vi "SP.vi"   [LabVIEW 2016]
uses:
  <vilib>/ULx/Create Channel.llb/ULx Create Channel (AI-Voltage-Basic).vi
  <vilib>/ULx/Timing.llb/ULx Timing (Sample Clock).vi
  <vilib>/ULx/Read.llb/ULx Read (Analog 1D Wfm NChan NSamp).vi
  <vilib>/Waveform/WDTOps.llb/WDT Index Channel DBL.vi
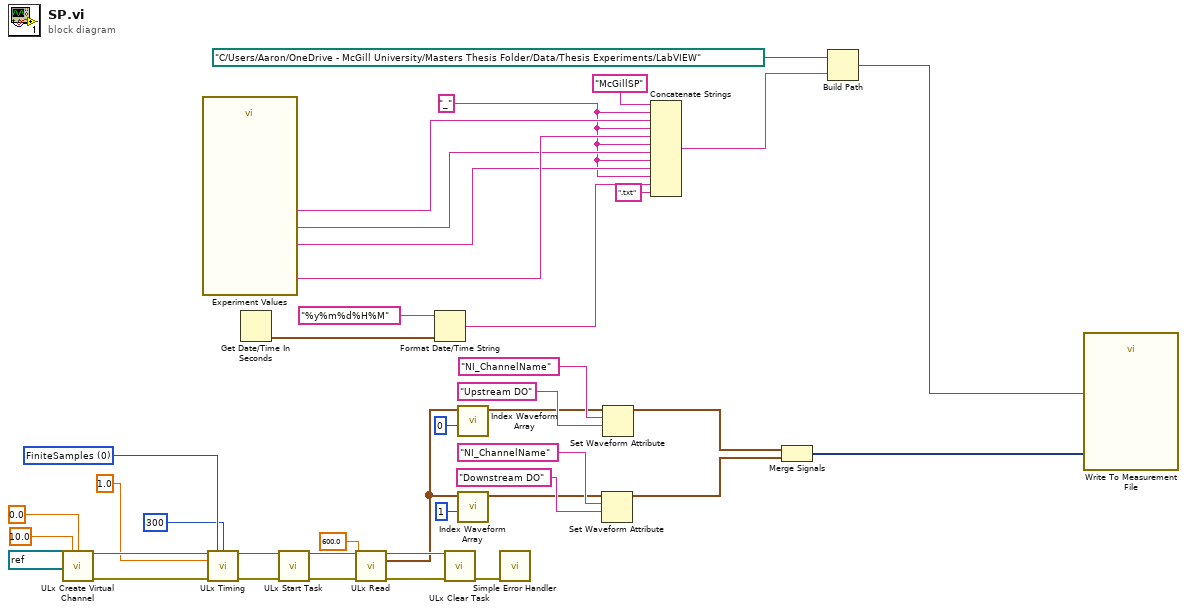
[diagram p0: block diagram]
diagram:
  w3 = "_"
  w29 = 0 items=["FiniteSamples", "ContinuousSamples"] ("sample mode")
  n1 = call-poly <vilib>:"ULx Create Virtual Channel.vi"("maximum value"=10.0, "minimum value"=0.0, "physical channels"=refnum<k21> "Dev0/Ai8:9") -> ("task out"=w41:refnum<k24>, "error out"=w37:errorcluster)  [unwired: 11 in]
  n2 = call "Experiment Values"() -> ("Air Content %"=w6:string, "Water Temperature (C)"=w4:string, "Atmospheric Air Pressure (kPa)"=w5:string, "Water Flowrate (gpm)"=w9:string)  [unwired: 14 in, 2 out]
  n3 = call-poly <vilib>:"ULx Timing.vi"("task in"=w41, "sample mode"=w29, "samples per channel"=300, "rate"=1.0, "error in"=w37) -> ("task out"=w40:refnum<k24>, "error out"=w36:errorcluster)  [unwired: 9 in]
  n4 = Get Date/Time In Seconds() -> (seconds since 1Jan1904=w12:timestamp)
  n5 = call <vilib>:"ULx Start Task.vi"("task in"=w40, "error in"=w36) -> ("task out"=w39:refnum<k24>, "error out"=w35:errorcluster)  [unwired: 12 in]
  n6 = call-poly <vilib>:"ULx Read.vi"("task in"=w39, "timeout"=600.0, "error in"=w35) -> ("task out"=w38:refnum<k24>, "data"=w25:waveform(dbl)[], "error out"=w34:errorcluster)  [unwired: 10 in]
  n7 = Format Date/Time String(time format string (%c)="%y%m%d%H%M", seconds (now)=w12) -> (date/time string=w2:string)  [unwired: 1 in]
  n8 = call <vilib>:"ULx Clear Task.vi"("task in"=w38, "error in"=w34) -> ("error out"=w33:errorcluster)  [unwired: 13 in]
  n9 = call-poly <vilib>:"Index Waveform Array.vi"("index"=0, "waveform array"=w25) -> ("waveform"=w22:waveform(dbl))  [unwired: 8 in, 1 out]
  n10 = call-poly <vilib>:"Index Waveform Array.vi"("index"=1, "waveform array"=w25) -> ("waveform"=w19:waveform(dbl))  [unwired: 8 in, 1 out]
  n11 = call <vilib>:"Simple Error Handler.vi"("error in (no error)"=w33) -> ()  [unwired: 4 in, 5 out]
  n12 = Set Waveform Attribute(5:"Downstream DO", 6:"NI_ChannelName" ("name"), 7:w19) -> (3:w17:waveform(dbl))  [unwired: 1 in, 2 out]
  n13 = Set Waveform Attribute(5:"Upstream DO", 6:"NI_ChannelName" ("name"), 7:w22) -> (3:w18:waveform(dbl))  [unwired: 1 in, 2 out]
  n14 = Concatenate Strings("McGillSP", w3, w9, w3, w6, w3, w5, w3, w4, w3, w2, ".txt" ("string")) -> (w13:string)
  n15 = Merge Signals(w18, w17) -> (w16:dynamicdata)
  n16 = Build Path(base path=path "C:/Users/Aaron/OneDrive - McGill University/Masters Thesis Folder/Data/Thesis Experiments/LabVIEW" ("Filename"), name or relative path=w13) -> (appended path=w14:path)
  n17 = call "Write To Measurement File"("Signals"=w16, "Filename"=w14) -> ()  [unwired: 15 in, 3 out]
